vi "Get Gyro Angle.vi"() -> (0 "Angle":dbl)   [LabVIEW 2012]
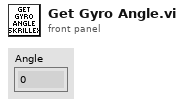
[diagram p1: front panel]
types:
  T1 = typedef "WPI_DigitalInputDevRef.ctl" = cluster{"DevStatus":errorcluster, "DIO Channel":T2, "Digital Module":T3}
  T2 = typedef "FPGA_DIOChannel.ctl" = enum8{"DIO 1", "DIO 2", "DIO 3", "DIO 4", "DIO 5", "DIO 6", "DIO 7", "DIO 8", "DIO 9", "DIO 10", "DIO 11", "DIO 12", "DIO 13", "DIO 14", "Invalid"}
  T3 = typedef "FPGA_TypedefDigitalModule.ctl" = enum16{"Digital Module 1", "Digital Module 2"}
  T4 = typedef "WPI_GyroDevRef.ctl" = cluster{"DevStatus":errorcluster, "Analog Module":T5, "Analog Channel":T6, "Offset":dbl, "Gain (VoltsPerDegree/Second)":dbl}
  T5 = typedef "FPGA_TypedefAnalogModule.ctl" = enum16{"Analog Module 1", "Analog Module 2"}
  T6 = typedef "FPGA_AIChannel.ctl" = enum8{"AI 1", "AI 2", "AI 3", "AI 4", "AI 5", "AI 6", "AI 7", "AI 8", "Invalid"}
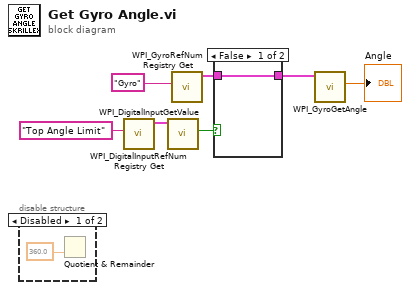
[diagram p0: block diagram]
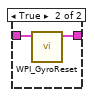
[diagram p3: hidden frame]
diagram:
  n1 = disable-structure shown="Disabled" {
    frame Disabled {
      n2 = Quotient & Remainder(y=360.0) -> ()  [unwired: 1 in, 2 out]
    }
    frame Enabled {
    }
  }
  n3 = call <vilib>:"WPI_DigitalInputRefNum Registry Get.vi"("refnum name"="Top Angle Limit") -> ("DigitalInputDevRef"=w5:T1)  [unwired: 9 in, 1 out]
  n4 = call <vilib>:"WPI_DigitalInputGetValue.vi"("DigitalInputDevRef"=w5) -> ("Value"=w2:bool)  [unwired: 8 in, 2 out]
  n5 = call <vilib>:"WPI_GyroRefNum Registry Get.vi"("refnum name"="Gyro") -> ("GyroDevRef"=w4:T4)  [unwired: 9 in, 1 out]
  n6 = case shown="False" w2 {
    tunnel: w4 -> [w9 w11]
    tunnel: [w9 w10] -> w7
    frame False {
    }
    frame True {
      n7 = call <vilib>:"WPI_GyroReset.vi"("GyroDevRef"=w11) -> ("GyroDevRef"=w10:T4)  [unwired: 9 in, 1 out]
    }
  }
  n8 = call <vilib>:"WPI_GyroGetAngle.vi"("GyroDevRef"=w7) -> ("Angle"=→"Angle":dbl)  [unwired: 7 in, 3 out]
